vi "Create Request Object.vi"(1 "Notification?":bool, 2 "params":variant, 3 "method":string) -> (0 "request":T1)   [LabVIEW 2019, in "JSON-RPC.lvclass"]
uses:
  JSON-RPC.lvclass
  typedefs/Request--Cluster.ctl
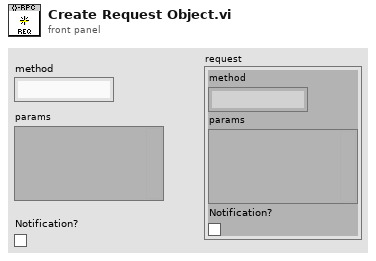
[diagram p1: front panel]
types:
  T1 = typedef "JSON-RPC.lvclass/Request--Cluster.ctl" = cluster{"method":string, "params":variant, "Notification?":bool}
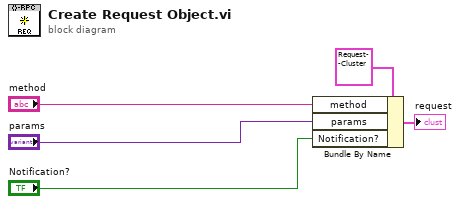
[diagram p0: block diagram]
diagram:
  n1 = Bundle By Name(cluster=T1 {"method"="", "params"=variant, "Notification?"=FALSE} ("request"), "method"="method", "params"="params", "Notification?"="Notification?") -> (→"request":T1)
